vi "SFID_Convert serial string to Eng vals.vi"(1 "Serial buffer string (excluding FrameChar)":string) -> (0 "SFID data":T1)   [LabVIEW 2022 SP3]
uses:
  Ctls/SFID_Data.ctl
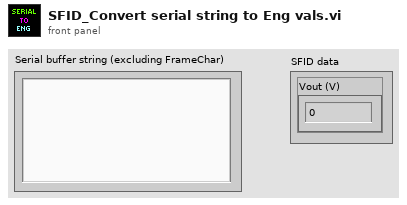
[diagram p1: front panel]
types:
  T1 = typedef "SFID_Data.ctl" = cluster{"Vout (V)":sgl}
  T2 = enum16{"big-endian, network order", "native, host order", "little-endian"}
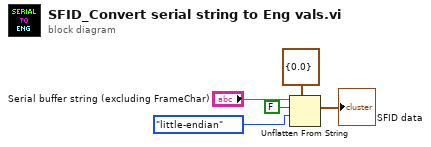
[diagram p0: block diagram]
diagram:
  n1 = Unflatten From String(type=T1 {"Vout (V)"=0.0} ("R_isol module data"), binary string="Serial buffer string (excluding FrameChar)", data includes array or string size? (T)=FALSE, byte order (0:big-endian, network order)=T2."little-endian") -> (value=→"SFID data":T1)  [unwired: 1 in, 2 out]
